vi "GigE Vision Set Socket Buffer Size.vi"(8 "error in (no error)":errorcluster, 10 "Buffer Size":u32, 11 "Camera in":refnum<class "Camera.lvclass">) -> (0 "error out":errorcluster, 3 "Camera":refnum<class "Camera.lvclass">)   [LabVIEW 2020, in "Camera.lvclass"]
uses:
  Camera.lvclass
  Camera.lvclass/Camera.ctl
  bin/gindustrialcam_32-1.dll
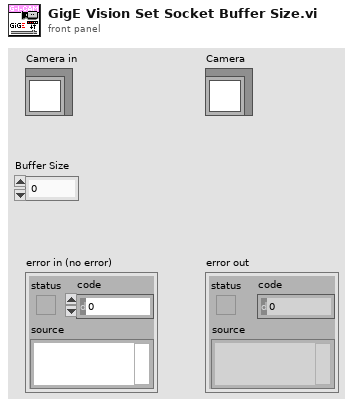
[diagram p1: front panel]
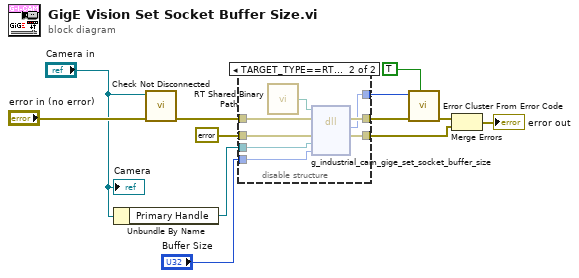
[diagram p0: block diagram]
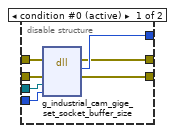
[diagram p2: hidden frame]
diagram:
  n1 = Unbundle By Name("Camera in") -> ("Primary Handle"=w2:refnum<data-value>)
  n2 = call "Check Not Disconnected.vi"("error in (no error)"="error in (no error)", "Camera in"="Camera in") -> ("error out"=w10:errorcluster)  [unwired: 9 in]
  n3 = disable-structure shown="TARGET_TYPE==RT&&OS==Linux" {
    disable-tunnel: w10 -> [w19 w27]
    disable-tunnel: errorcluster {"status"=FALSE, "code"=0, "source"=""} ("error constant") -> [w18 w25]
    disable-tunnel: [w17 w22] -> w7
    disable-tunnel: [w16 w23] -> w5
    disable-tunnel: [w15 w24] -> w4
    disable-tunnel: w2 -> [w14 w21]
    disable-tunnel: "Buffer Size" -> [w13 w20]
    frame condition #0 (active) {
      n4 = dll-call lib="C:/serenial/lib/g-industrial-camera/LabVIEW/g_industrial_cam/bin/gindustrialcam_*-1.*" fn="g_industrial_cam_gige_set_socket_buffer_size"(error in=w19, "err"=w18, "edvr"=w14, "buffer size"=w13) -> (error out=w15:errorcluster, "Mg_Error"=w16:i32, "err"=w17:errorcluster)  [unwired: 4 in, 1 out]
    }
    frame condition #1 {
      n5 = call "RT Shared Binary Path.vi"() -> ("Path"=w26:path)
      n6 = dll-call lib="?" fn="g_industrial_cam_gige_set_socket_buffer_size"(path in=w26, error in=w27, "err"=w25, "edvr"=w21, "buffer size"=w20) -> (error out=w24:errorcluster, "Mg_Error"=w23:i32, "err"=w22:errorcluster)  [unwired: 3 in, 1 out]
    }
  }
  n7 = call <vilib>:"Error Cluster From Error Code.vi"("show call chain? (False)"=TRUE, "error in (no error)"=w4, "error code (0)"=w5) -> ("error out"=w6:errorcluster)  [unwired: 6 in]
  n8 = Merge Errors(w6, w7) -> (→"error out":errorcluster)
  "Camera" <- "Camera in"
